vi "Viewer.vi"(8 "error in (no error)":errorcluster, 9 "StopAcq":refnum<notifier>, 10 "Stop":refnum<notifier>, 11 "TopicQ":refnum<queue>) -> (0 "error out":errorcluster)   [LabVIEW 2018, in "TopicViewer.lvlib"]
uses:
  TopicViewer.lvlib
panel:
  in  "Local Stop":bool
  out "Console":string
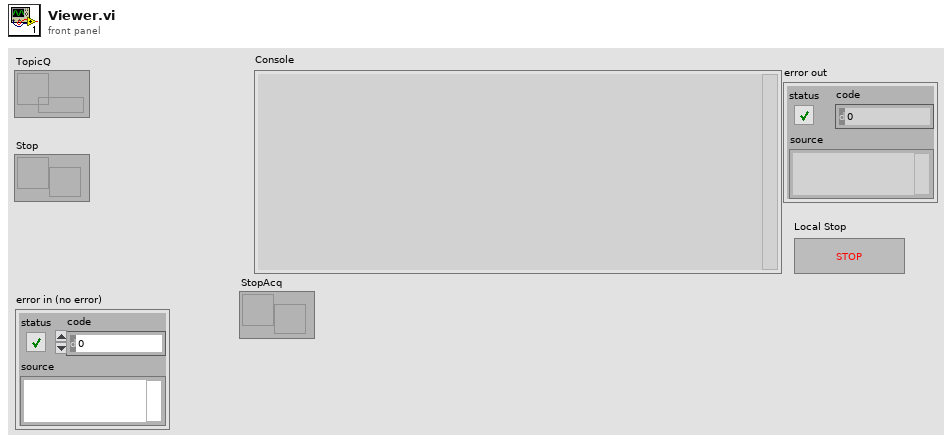
[diagram p1: front panel]
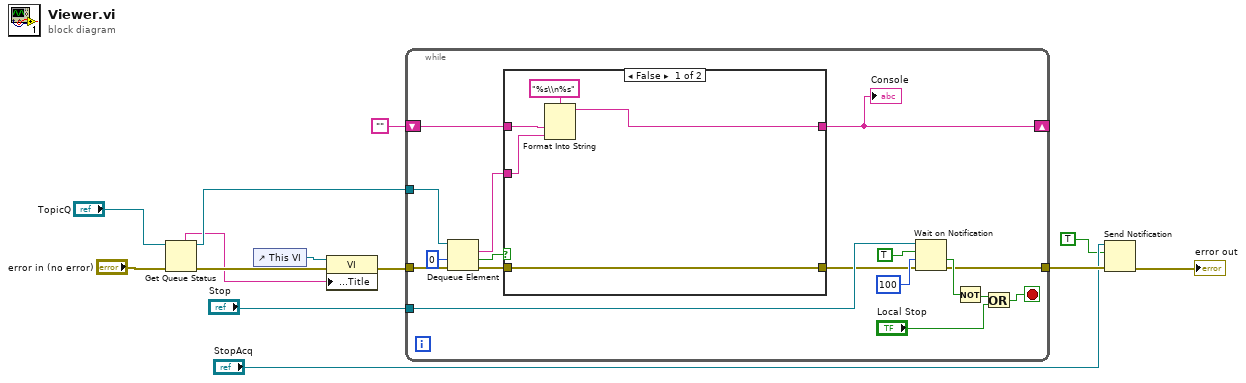
[diagram p0: block diagram]
diagram:
  n1 = Get Queue Status(queue="TopicQ", error in (no error)="error in (no error)") -> (queue out=w6:refnum<queue>, queue name=w1:string, error out=w2:errorcluster)  [unwired: 1 in, 5 out]
  n2 = control-ref of="This VI"() -> (w3:refnum<vi>)
  n3 = property class="VI"(reference=w3, error in=w2, "Front Panel.Title"=w1) -> (error out=w4:errorcluster)  [unwired: 1 out]
  n4 = while {
    tunnel: w6 -> [w26]
    tunnel: "Stop" -> [w30]
    tunnel: w4 -> [w25]
    shift-right: [w17] -> _
    shift-left: "" -> [w18]
    tunnel: [w19] -> w11
    stop <- w14 stop-if-true
    n5 = Dequeue Element(queue=w26, timeout in ms (-1)=0, error in (no error)=w25) -> (element=w21:string, timed out?=w23:bool, error out=w24:errorcluster)  [unwired: 1 out]
    n6 = case shown="False" w23 {
      tunnel: w24 -> [w35 w36]
      tunnel: w21 -> [w33 _]
      tunnel: [w35 w36] -> w20
      tunnel: w18 -> [w32 w37]
      tunnel: [w31 w37] -> w17
      frame False {
        n7 = Format Into String(format string="%s\\n%s", w32, w33) -> (resulting string=w31:string)  [unwired: 2 in, 1 out]
      }
      frame True {
      }
    }
    "Console" <- w17
    n8 = Wait on Notification(notifier=w30, ignore previous (F)=TRUE, timeout in ms (-1)=100, error in (no error)=w20) -> (timed out?=w29:bool, error out=w19:errorcluster)  [unwired: 2 out]
    n9 = Not(x=w29) -> (.not. x?=w16:bool)
    n10 = Or(x=w16, y="Local Stop") -> (x .or. y?=w14:bool)
  }
  n11 = Send Notification(notification=TRUE, notifier="StopAcq", error in (no error)=w11) -> (error out=→"error out":errorcluster)  [unwired: 1 out]
